vi "Get Image Timings.vi"(8 "error in (no error)":errorcluster, 11 "Save Image in":refnum<class "Save Image.lvclass">) -> (0 "error out":errorcluster, 3 "Save Image out":refnum<class "Save Image.lvclass">)   [LabVIEW 2018, in "Save Image.lvclass"]
uses:
  Save Image.lvclass
  Save Image.lvclass/Save Image.ctl
  Interface/Interface.lvclass/Interface.ctl
  Interface/Interface.lvclass
  Simulated_Header/Simulated_Header.lvclass
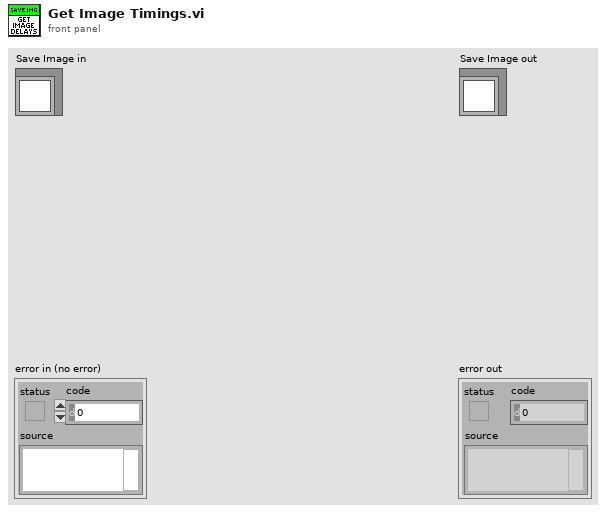
[diagram p1: front panel]
types:
  T1 = cluster{"COOLER_POWER_STATUS":u16, "TEMP":i32, "EXPTIME":dbl, "#FRAMES":u32, "#CUBES":u32}
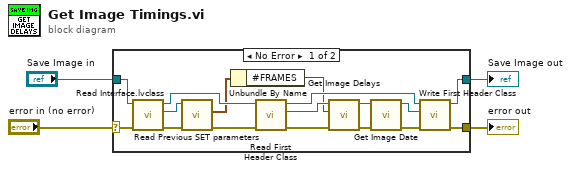
[diagram p0: block diagram]
diagram:
  n1 = case shown="No Error" "error in (no error)" {
    selector: "error in (no error)" -> [w15 w23]
    tunnel: [w20 w23] -> w3
    tunnel: [w21 w22] -> w1
    tunnel: "Save Image in" -> [w16 w22]
    frame No Error {
      n2 = call "Read Interface.lvclass.vi"("error in (no error)"=w15, "Save Image in"=w16) -> ("error out"=w10:errorcluster, "Interface.lvclass"=w11:refnum<class "Interface.lvclass">, "Save Image out"=w14:refnum<class "Save Image.lvclass">)  [unwired: 7 in]
      n3 = call "Read Previous SET parameters.vi"("error in (no error)"=w10, "Interface in"=w11) -> ("error out"=w9:errorcluster, "Previous SET parameters"=w13:T1)  [unwired: 7 in, 1 out]
      n4 = Unbundle By Name(w13) -> ("#FRAMES"=w12:u32)
      n5 = call "Read First Header Class.vi"("error in (no error)"=w9, "Save Image in"=w14) -> ("error out"=w17:errorcluster, "Simulated_Header.lvclass"=w19:refnum<class "Simulated_Header.lvclass">, "Save Image out"=w18:refnum<class "Save Image.lvclass">)  [unwired: 7 in]
      n6 = call-dynamic "Get Image Delays.vi"("error in (no error)"=w17, "frames"=w12, "Simulated_Header in"=w19) -> ("error out"=w5:errorcluster, "Simulated_Header out"=w8:refnum<class "Simulated_Header.lvclass">)  [unwired: 7 in]
      n7 = call-dynamic "Get Image Date.vi"("error in (no error)"=w5, "Simulated_Header in"=w8) -> ("error out"=w6:errorcluster, "Simulated_Header out"=w7:refnum<class "Simulated_Header.lvclass">)  [unwired: 8 in]
      n8 = call "Write First Header Class.vi"("error in (no error)"=w6, "Simulated_Header.lvclass"=w7, "Save Image in"=w18) -> ("error out"=w20:errorcluster, "Save Image out"=w21:refnum<class "Save Image.lvclass">)  [unwired: 7 in]
    }
    frame Error {
    }
  }
  "error out" <- w3
  "Save Image out" <- w1
